vi "getGlyphFile.vi"(8 "error in (no error)":errorcluster, 11 "Channel_FXP in":refnum<class "Channel_FXP.lvclass">) -> (0 "error out":errorcluster, 2 "Glyph File":string, 3 "Channel_FXP out":refnum<class "Channel_FXP.lvclass">)   [LabVIEW 2013, in "Channel_FXP.lvclass"]
doc: "Dynamic Dispatch VI. Returns the name of the glyph file to be used as a glyph in the tree control. A empty string means no glyph."
uses:
  Channel_FXP.lvclass
  Channel/Channel.lvclass
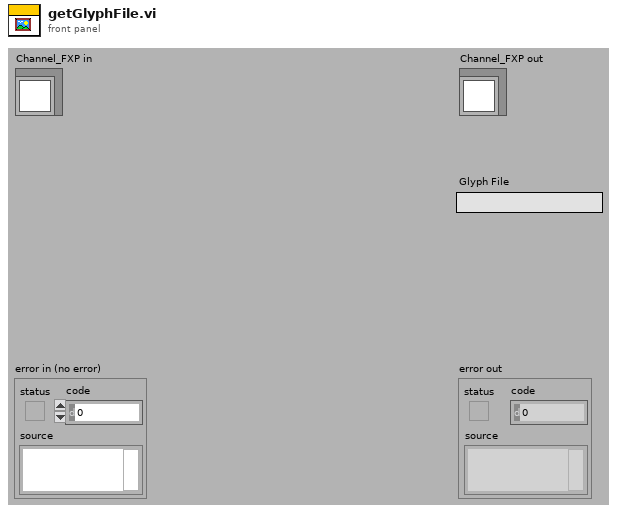
[diagram p1: front panel]
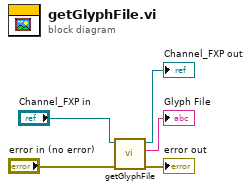
[diagram p0: block diagram]
diagram:
  n1 = call-parent "getGlyphFile.vi"("error in (no error)"="error in (no error)", "Channel in"="Channel_FXP in") -> ("error out"=→"error out":errorcluster, "Glyph File"=→"Glyph File":string, "Channel out"=→"Channel_FXP out":refnum<class "Channel_FXP.lvclass">)  [unwired: 7 in]
